vi "Read Driver Setting Mappings.vi"(8 "error in (no error)":errorcluster, 11 "Driver in":refnum<class "Driver.lvclass">) -> (0 "error out":errorcluster, 2 "Driver Setting Mappings":T1[](array[typedef]), 3 "Driver out":refnum<class "Driver.lvclass">)   [LabVIEW 2023, in "HAF.lvlib" / "Driver.lvclass"]
doc: "Returns the current set of Driver Setting mappings. Builds this if an empty array."
uses:
  Driver.lvclass
  Driver.lvclass/Driver.ctl
  Setting Map Structure.ctl
  HAF.lvlib
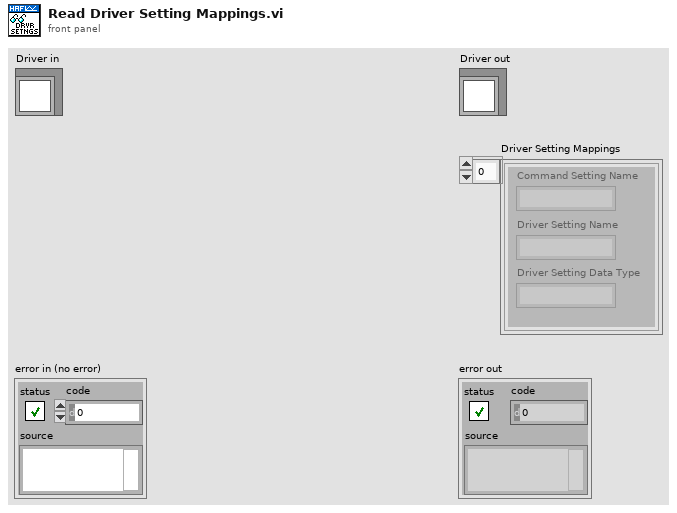
[diagram p1: front panel]
types:
  T1 = typedef "HAF.lvlib/Setting Map Structure.ctl" = cluster{"Command Setting Name":string, "Driver Setting Name":string, "Driver Setting Data Type":string}
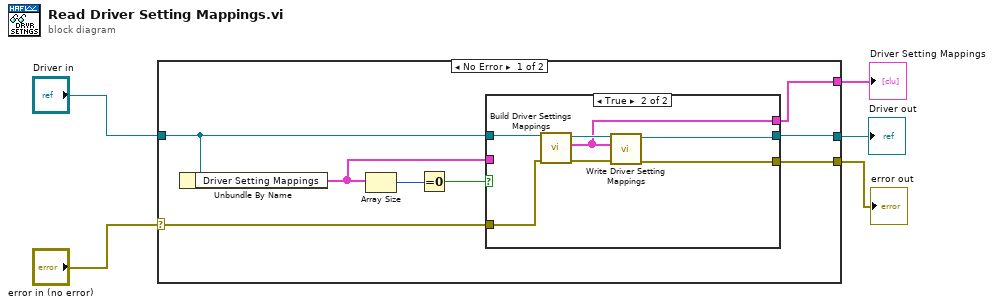
[diagram p0: block diagram]
diagram:
  n1 = case shown="No Error" "error in (no error)" {
    selector: "error in (no error)" -> [w9 w24]
    tunnel: [w7 w24] -> w4
    tunnel: [w8 w25] -> w2
    tunnel: "Driver in" -> [w11 w25]
    tunnel: [w6 _] -> w1
    frame No Error {
      n2 = Unbundle By Name(w11) -> ("Driver Setting Mappings"=w10:T1[])
      n3 = Array Size(array=w10) -> (size(s)=w13:i32)
      n4 = Equal To 0?(x=w13) -> (x = 0?=w12:bool)
      n5 = case shown="True" w12 {
        tunnel: w11 -> [w15 w23]
        tunnel: w10 -> [w16 _]
        tunnel: [w16 w18] -> w6
        tunnel: [w15 w19] -> w8
        tunnel: w9 -> [w14 w22]
        tunnel: [w14 w17] -> w7
        frame False {
        }
        frame True {
          n6 = call-dynamic "Build Driver Settings Mappings.vi"("error in (no error)"=w22, "Driver in"=w23) -> ("error out"=w20:errorcluster, "Array"=w18:T1[], "Driver out"=w21:refnum<class "Driver.lvclass">)  [unwired: 7 in]
          n7 = call-dynamic "Write Driver Setting Mappings.vi"("error in (no error)"=w20, "Driver Setting Mappings"=w18, "Driver in"=w21) -> ("error out"=w17:errorcluster, "Driver out"=w19:refnum<class "Driver.lvclass">)  [unwired: 7 in]
        }
      }
    }
    frame Error {
    }
  }
  "error out" <- w4
  "Driver out" <- w2
  "Driver Setting Mappings" <- w1
